vi "Read Window Position and Size.vi"(8 "error in":errorcluster, 10 "Position Key":string, 11 "VI Refnum":refnum<vi>) -> (0 "error out":errorcluster)   [LabVIEW 2019, in "Shared.lvlib"]
uses:
  Shared.lvlib
  <vilib>/Utility/miscctls.llb/LVRectTypeDef.ctl
  <vilib>/Utility/config.llb/Read Key (String).vi
  <vilib>/Utility/config.llb/NI_LVConfig.lvlib
  Panther Dashboard/Panther Dashboard.lvlib
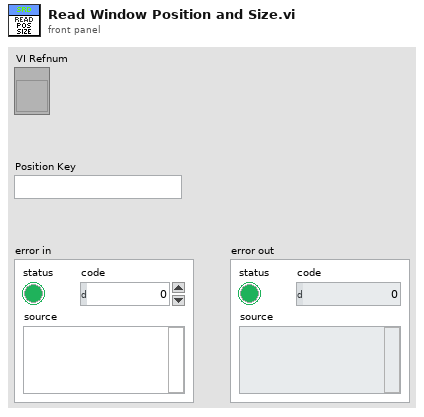
[diagram p1: front panel]
types:
  T1 = typedef "LVRectTypeDef.ctl" = cluster{"Left":i16, "Top":i16, "Right":i16, "Bottom":i16}
  T2 = typedef "NI_LVConfig.lvlib/Config Data RefNum.ctl" = refnum<k1>
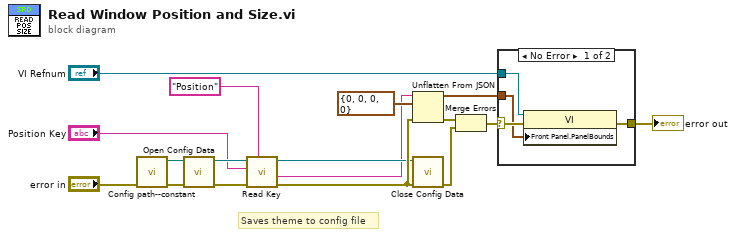
[diagram p0: block diagram]
diagram:
  # "Saves theme to config file"
  n1 = call "Config path--constant.vi"("error in (no error)"="error in") -> ("error out"=w15:errorcluster, "Config Path"=w5:path)  [unwired: 9 in]
  n2 = call <vilib>:"Open Config Data.vi"("error in (no error)"=w15, "configuration file path"=w5) -> ("error out"=w16:errorcluster, "refnum"=w8:T2)  [unwired: 7 in, 1 out]
  n3 = call-poly <vilib>:"Read Key.vi"("section"="Position", "error in (no error)"=w16, "key"="Position Key", "refnum"=w8) -> ("error out"=w10:errorcluster, "value"=w3:string, "refnum out"=w9:T2)  [unwired: 4 in, 1 out]
  n4 = Unflatten From JSON(JSON string=w3, type and defaults=T1 {"Left"=0, "Top"=0, "Right"=0, "Bottom"=0} ("NewBnds"), error in (no error)=w10) -> (value=w1:T1, error out=w13:errorcluster)  [unwired: 4 in]
  n5 = call <vilib>:"Close Config Data.vi"("error in (no error)"=w10, "refnum"=w9) -> ("error out"=w17:errorcluster)  [unwired: 8 in, 1 out]
  n6 = Merge Errors(w13, w17) -> (w11:errorcluster)
  n7 = case shown="No Error" w11 {
    selector: w11 -> [w20 w22]
    tunnel: "VI Refnum" -> [w19 _]
    tunnel: [w21 w22] -> w12
    tunnel: w1 -> [w18 _]
    frame No Error {
      n8 = property class="VI"(reference=w19, error in=w20, "Front Panel.PanelBounds"=w18) -> (error out=w21:errorcluster)  [unwired: 1 out]
    }
    frame Error {
    }
  }
  "error out" <- w12
